vi "Subvi line gating.vi"(6 "Reset":bool, 8 "Nmax lines":u64=1, 9 "Line clock change":bool) -> (1 "Line gating":bool)   [LabVIEW 2017]
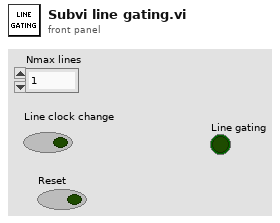
[diagram p1: front panel]
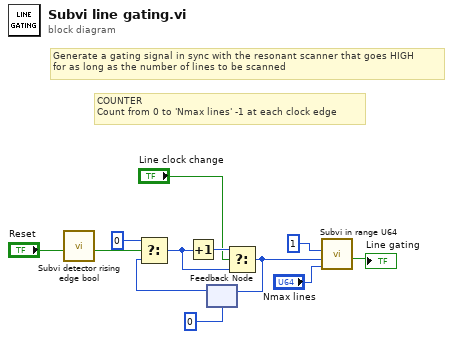
[diagram p0: block diagram]
diagram:
  # "COUNTER\nCount from 0 to 'Nmax lines' -1 at each clock edge"
  # "Generate a gating signal in sync with the resonant scanner that goes HIGH\nfor as long as the number of lines to be scanned"
  n1 = call "Subvi detector rising edge bool.vi"("Input"="Reset") -> ("Output"=w2:bool)  [unwired: 10 in]
  n2 = feedback #1(u64 0 ("t")) -> (w6:u64)
  n3 = Select(t=u64 0, s=w2, f=w6) -> (s? t:f=w3:u64)
  n4 = Increment(x=w3) -> (x+1=w12:u64)
  n5 = Select(t=w12, s="Line clock change", f=w3) -> (s? t:f=w7:u64)
  n6 = feedback-in #1(w7) -> ()
  n7 = call "Subvi in range U64.vi"("Max"="Nmax lines", "Input"=w7, "Min"=u64 1) -> ("In range"=→"Line gating":bool)  [unwired: 8 in]
